vi "Read (Single Point).vi"(8 "error in (no error)":errorcluster, 11 "VISA resource name":refnum<visa-resource-name>) -> (0 "error out":errorcluster, 2 "Measurement":dbl, 3 "VISA resource name out":refnum<visa-resource-name>)   [LabVIEW 2013, in "Template - DMM.lvlib"]
doc: "Reads and returns a single measurement from the instrument."
uses:
  <instrlib>/_Template - DMM/Template - DMM.lvlib
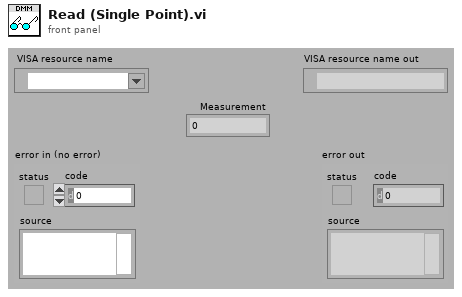
[diagram p1: front panel]
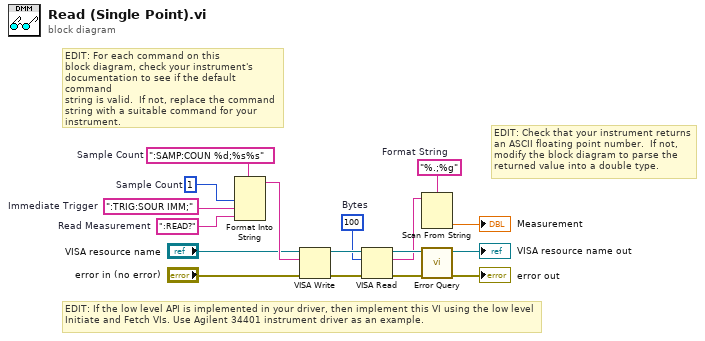
[diagram p0: block diagram]
diagram:
  w1 = 1  # Sample Count
  w5 = ":TRIG:SOUR IMM;"  # Immediate Trigger
  w7 = ":SAMP:COUN %d;%s%s"  # Sample Count
  w6 = ":READ?"  # Read Measurement
  w9 = "%.;%g"  # Format String
  w15 = u32 100  # Bytes
  # "EDIT: If the low level API is implemented in your driver, then implement this VI using the low level Initiate and Fetch VIs. Use Agilent 34401 instrument driver as an example."
  # "EDIT: Check that your instrument returns\nan ASCII floating point number.  If not, \nmodify the block diagram to parse the\nreturned value into a double type."
  # "EDIT: For each command on this\nblock diagram, check your instrument's\ndocumentation to see if the default command\nstring is valid.  If not, replace the command\nstring with a suitable command for your\ninstrument."
  n1 = Format Into String(format string=w7, w1, w5, w6) -> (resulting string=w4:string)  [unwired: 2 in, 1 out]
  n2 = VISA Write(VISA resource name="VISA resource name", write buffer=w4, error in (no error)="error in (no error)") -> (VISA resource name out=w16:refnum<visa-resource-name>, error out=w17:errorcluster)  [unwired: 1 out]
  n3 = VISA Read(VISA resource name=w16, byte count=w15, error in (no error)=w17) -> (VISA resource name out=w14:refnum<visa-resource-name>, read buffer=w10:string, error out=w13:errorcluster)  [unwired: 1 out]
  n4 = Scan From String(format string=w9, input string=w10) -> (output 1=→"Measurement":dbl)  [unwired: 3 in, 3 out]
  n5 = call <instrlib>:"Error Query.vi"("error in (no error)"=w13, "VISA resource name"=w14) -> ("error out"=→"error out":errorcluster, "VISA resource name out"=→"VISA resource name out":refnum<visa-resource-name>)  [unwired: 6 in, 2 out]
